vi "Attach Params to URL.vi"(8 "Error in":errorcluster caption="Error in (no error)", 10 "URL":string, 11 "Param array":T1[](array[typedef])) -> (0 "Error out":errorcluster, 2 "URL with params":string)   [LabVIEW 2018]
uses:
  TypeDef/Param.ctl
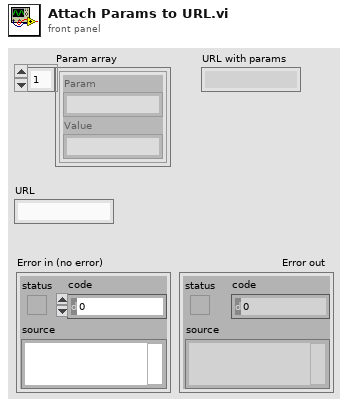
[diagram p1: front panel]
types:
  T1 = typedef "Param.ctl" = cluster{"Param":string, "Value":string}
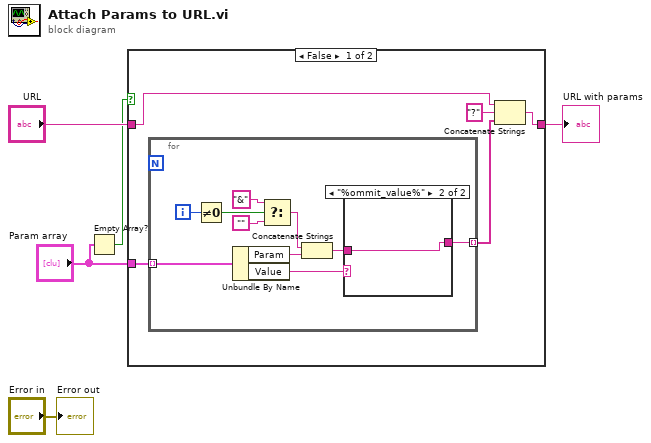
[diagram p0: block diagram]
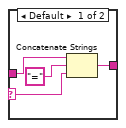
[diagram p2: hidden frame]
diagram:
  n1 = Empty Array?(array="Param array") -> (empty?=w3:bool)
  n2 = case shown="False" w3 {
    tunnel: "Param array" -> [w10 _]
    tunnel: "URL" -> [w9 w26]
    tunnel: [w8 w26] -> w5
    frame False {
      n3 = for {
        tunnel: w10 -> [w20] mode=indexing
        tunnel: [w11] -> w6 mode=indexing
        i -> [w19]
        n4 = Not Equal To 0?(x=w19) -> (x != 0?=w18:bool)
        n5 = Unbundle By Name(w20) -> ("Param"=w14:string, "Value"=w13:string)
        n6 = Select(t="&" ("string"), s=w18, f="") -> (s? t:f=w15:string)
        n7 = Concatenate Strings(w15, w14) -> (w12:string)
        n8 = case shown="\"%ommit_value%\"" w13 {
          selector: w13 -> [w22 _]
          tunnel: [w23 w25] -> w11
          tunnel: w12 -> [w21 w25]
          frame Default {
            n9 = Concatenate Strings(w21, "=" ("string"), w22) -> (w23:string)
          }
          frame "%ommit_value%" {
          }
        }
      }
      n10 = Concatenate Strings(w9, "?" ("string"), w6) -> (w8:string)
    }
    frame True {
      # "No Params to attach"
    }
  }
  "URL with params" <- w5
  "Error out" <- "Error in"
